vi "Get Hardware Configuration File Path.vi"(8 "error in":errorcluster, 11 "Ballard ARINC 429 custom device in":T1 format="%.0x") -> (0 "error out":errorcluster, 1 "RT destination":path, 2 "hardware configuration file path":path, 3 "Ballard ARINC 429 custom device out":T1 format="%.0x")   [LabVIEW 2020, in "AIM ARINC 429 Scripting.lvlib"]
doc: "Returns the <b>hardware configuration file path</b>. The hardware configuration file must be consistent with system configuration for successful deployment and avionics bus communication."
uses:
  AIM ARINC 429 Scripting.lvlib
  <vilib>/NI VeriStand/Custom Device API/Custom Device Item Ref.ctl
  Constants.vi
  <vilib>/NI VeriStand/Custom Device API/Get Item Property (Dependent File).vi
  <vilib>/NI VeriStand/Custom Device API/Custom Device API.lvlib
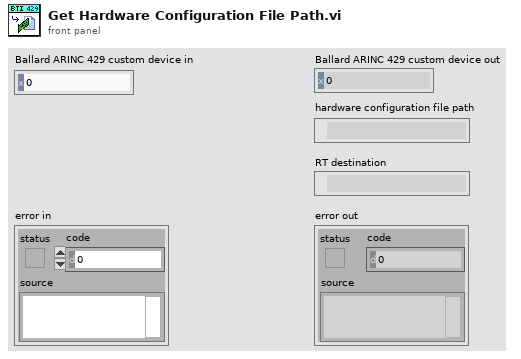
[diagram p1: front panel]
types:
  T1 = typedef "Custom Device API.lvlib/Custom Device Item Ref.ctl" = u64
  T2 = typedef "Custom Device API.lvlib/Dependent File Optional Info.ctl" = cluster{"Version":string, "RTDestination":path, "ForceDownload":bool, "SupportedTarget":string, "MD5":string}
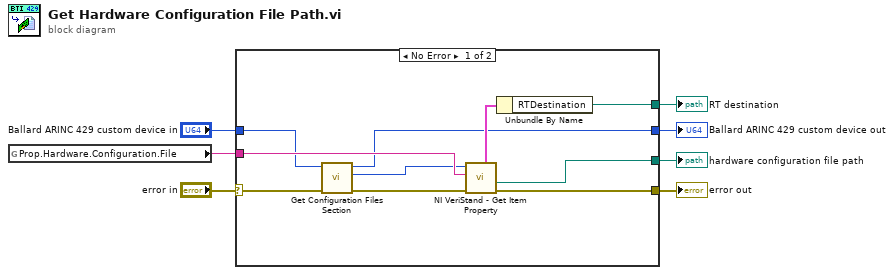
[diagram p0: block diagram]
diagram:
  n1 = global read "Constants.vi" "Prop.Hardware.Configuration.File"() -> (w1:string)
  n2 = case shown="No Error" "error in" {
    selector: "error in" -> [w12 w19]
    tunnel: "Ballard ARINC 429 custom device in" -> [w9 w18]
    tunnel: [w16 w19] -> w6
    tunnel: [w8 w18] -> w4
    tunnel: [w17 _] -> w3
    tunnel: [w14 _] -> w2
    tunnel: w1 -> [w13 _]
    frame No Error {
      n3 = call "Get Configuration Files Section.vi"("error in"=w12, "Custom device Ref"=w9) -> ("error out"=w11:errorcluster, "Configuration files Ref"=w10:T1, "Custom device Ref out"=w8:T1)  [unwired: 7 in]
      n4 = call-poly <vilib>:"NI VeriStand - Get Item Property.vi"("error in (no error)"=w11, "Property Name"=w13, "Item Ref in"=w10) -> ("error out"=w16:errorcluster, "Path"=w17:path, "OptionalInfo"=w15:T2)  [unwired: 4 in, 2 out]
      n5 = Unbundle By Name(w15) -> ("RTDestination"=w14:path)
    }
    frame Error {
    }
  }
  "error out" <- w6
  "hardware configuration file path" <- w3
  "Ballard ARINC 429 custom device out" <- w4
  "RT destination" <- w2
